vi "Read PC SN.vi"(8 "error in (no error)":errorcluster) -> (0 "error out":errorcluster, 3 "Serial Number":string)   [LabVIEW 2017]
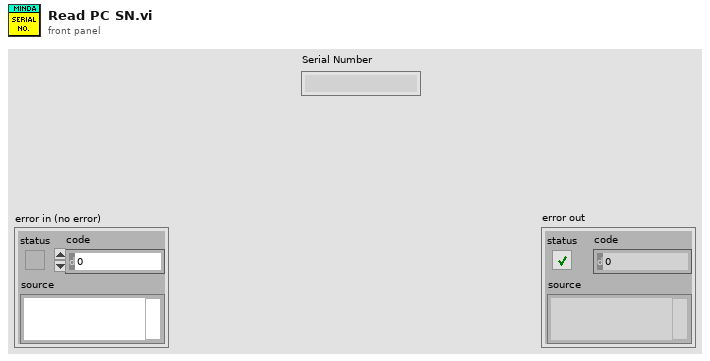
[diagram p1: front panel]
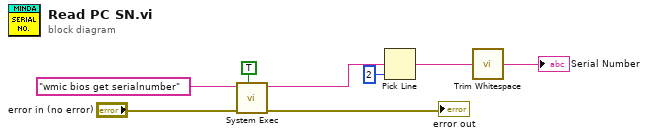
[diagram p0: block diagram]
diagram:
  n1 = call <vilib>:"System Exec.vi"("wait until completion? (T)"=TRUE ("run minimized? (F)"), "error in (no error)"="error in (no error)", "command line"="wmic bios get serialnumber") -> ("error out"=→"error out":errorcluster, "standard output"=w4:string)  [unwired: 5 in, 2 out]
  n2 = Pick Line(multi-line string=w4, line index=2) -> (output string=w2:string)  [unwired: 1 in]
  n3 = call <vilib>:"Trim Whitespace.vi"("string"=w2) -> ("trimmed string"=→"Serial Number":string)  [unwired: 1 in]
